vi "pf_Error_Codes_manager.vi"(7 "pf Error Type":T1, 8 "error in (no error)":errorcluster) -> (0 "error out":errorcluster, 3 "pf Error Code":i32)   [LabVIEW 2025, in "Photonfocus_Toolkit.lvlib"]
uses:
  Photonfocus_Toolkit.lvlib
  Controls/pf_Toolkit_Error_Type.ctl
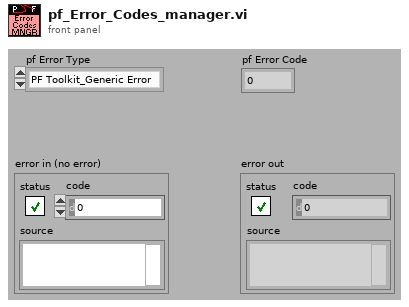
[diagram p1: front panel]
types:
  T1 = typedef "Photonfocus_Toolkit.lvlib/pf_Toolkit_Error_Type.ctl" = enum16{"PF Toolkit_Generic Error", "PF Toolkit_PFConfig Error"}
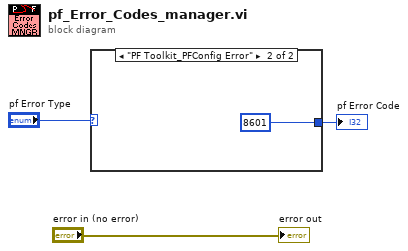
[diagram p0: block diagram]
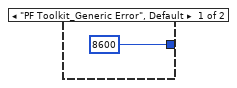
[diagram p2: hidden frame]
diagram:
  n1 = case shown="\"PF Toolkit_PFConfig Error\"" "pf Error Type" {
    tunnel: [8600 8601] -> w2
    frame "PF Toolkit_Generic Error", Default {
    }
    frame "PF Toolkit_PFConfig Error" {
    }
  }
  "pf Error Code" <- w2
  "error out" <- "error in (no error)"
